vi "Reset Buffer.vi"(11 "Block Upload Sub-Block Transfer in":refnum<class "Block Upload Sub-Block Transfer.lvclass">) -> (3 "Block Upload Sub-Block Transfer out":refnum<class "Block Upload Sub-Block Transfer.lvclass">)   [LabVIEW 2020, in "CANopen.lvlib" / "SDO Manager.lvlib" / "Block Upload Sub-Block Transfer.lvclass"]
uses:
  Block Upload Sub-Block Transfer.lvclass
  Block Upload Sub-Block Transfer.lvclass/Block Upload Sub-Block Transfer.ctl
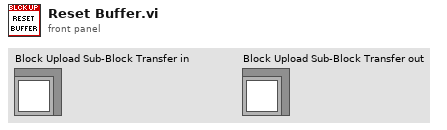
[diagram p1: front panel]
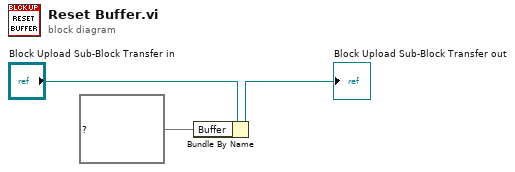
[diagram p0: block diagram]
diagram:
  n1 = Bundle By Name(cluster="Block Upload Sub-Block Transfer in", "Buffer"=map{u8, u8[]} {}) -> (→"Block Upload Sub-Block Transfer out":refnum<class "Block Upload Sub-Block Transfer.lvclass">)
